vi "Werte ändern (DBL_8xZ.I._Rechteck) (SubVI).vi"(0 "geladene Werte (Zeit (s); Wert)":dbl[][](array[numeric]), 1 "Zykluslänge":dbl, 2 "Z.I.":string, 3 "Info":string, 4 "Format+Namen":string) -> (5 "Ausgang":dbl[][](array[numeric]) format="%.2f", 6 "Z.I.":string, 7 "Sperre":bool)   [LabVIEW 2010]
panel:
  out "Fehlermeldung":string="Zeit ist größer als Zykluslänge"
  in  "löschen":bool
  out "aktuel 8":dbl
  out "aktuel 7":dbl
  out "aktuel 6":dbl
  out "aktuel 5":dbl
  out "aktuel 4":dbl
  out "aktuel 3":dbl
  out "aktuel2":dbl
  out "Name 8":string
  in  "Numerisch 8":dbl
  out "Name 7":string
  in  "Numerisch 7":dbl
  out "Name 6":string
  in  "Numerisch 6":dbl
  out "Name 5":string
  in  "Numerisch 5":dbl
  out "Name 4":string
  in  "Numerisch 4":dbl
  out "Name 3":string
  in  "Numerisch 3":dbl
  out "Name 2":string
  in  "Numerisch 2":dbl
  out "aktuel1":dbl
  out "Name 1":string
  in  "Numerisch 1":dbl
  out "aktuell (Zeit (s); Wert)":dbl[][](array[numeric])
  out "XY Graph":T1(graph) caption="XY-Graph"
  out "Zykluslänge":dbl format="%.2f"
  out "Info":string
  in  "neue Werte (Zeit (s); Wert)":dbl[][](array[numeric])
  in  "ändern":bool
  in  "zurück":bool
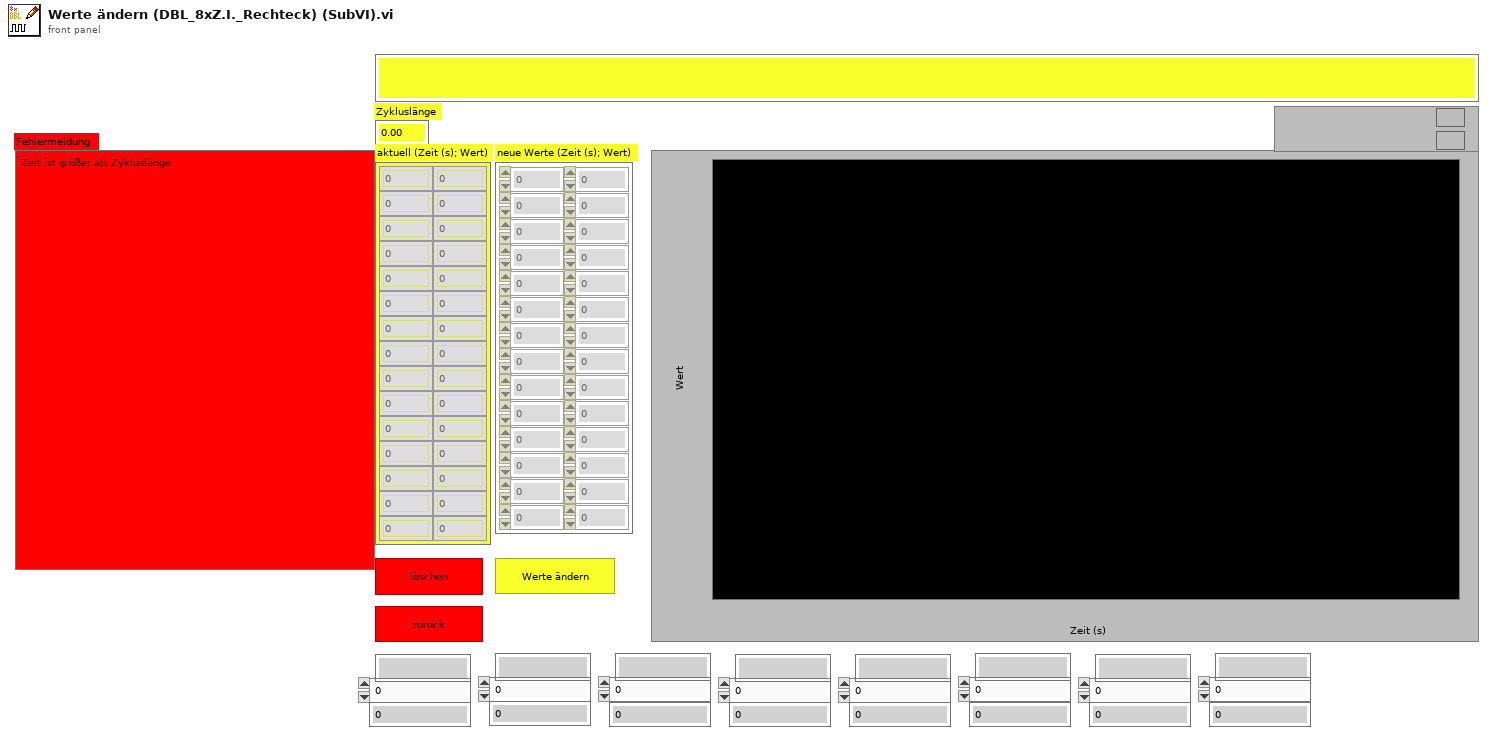
[diagram p1: front panel]
types:
  T1 = cluster{"neue Werte (Zeit (s); Wert)":dbl[], "neue Werte (Zeit (s); Wert)":dbl[]}[]
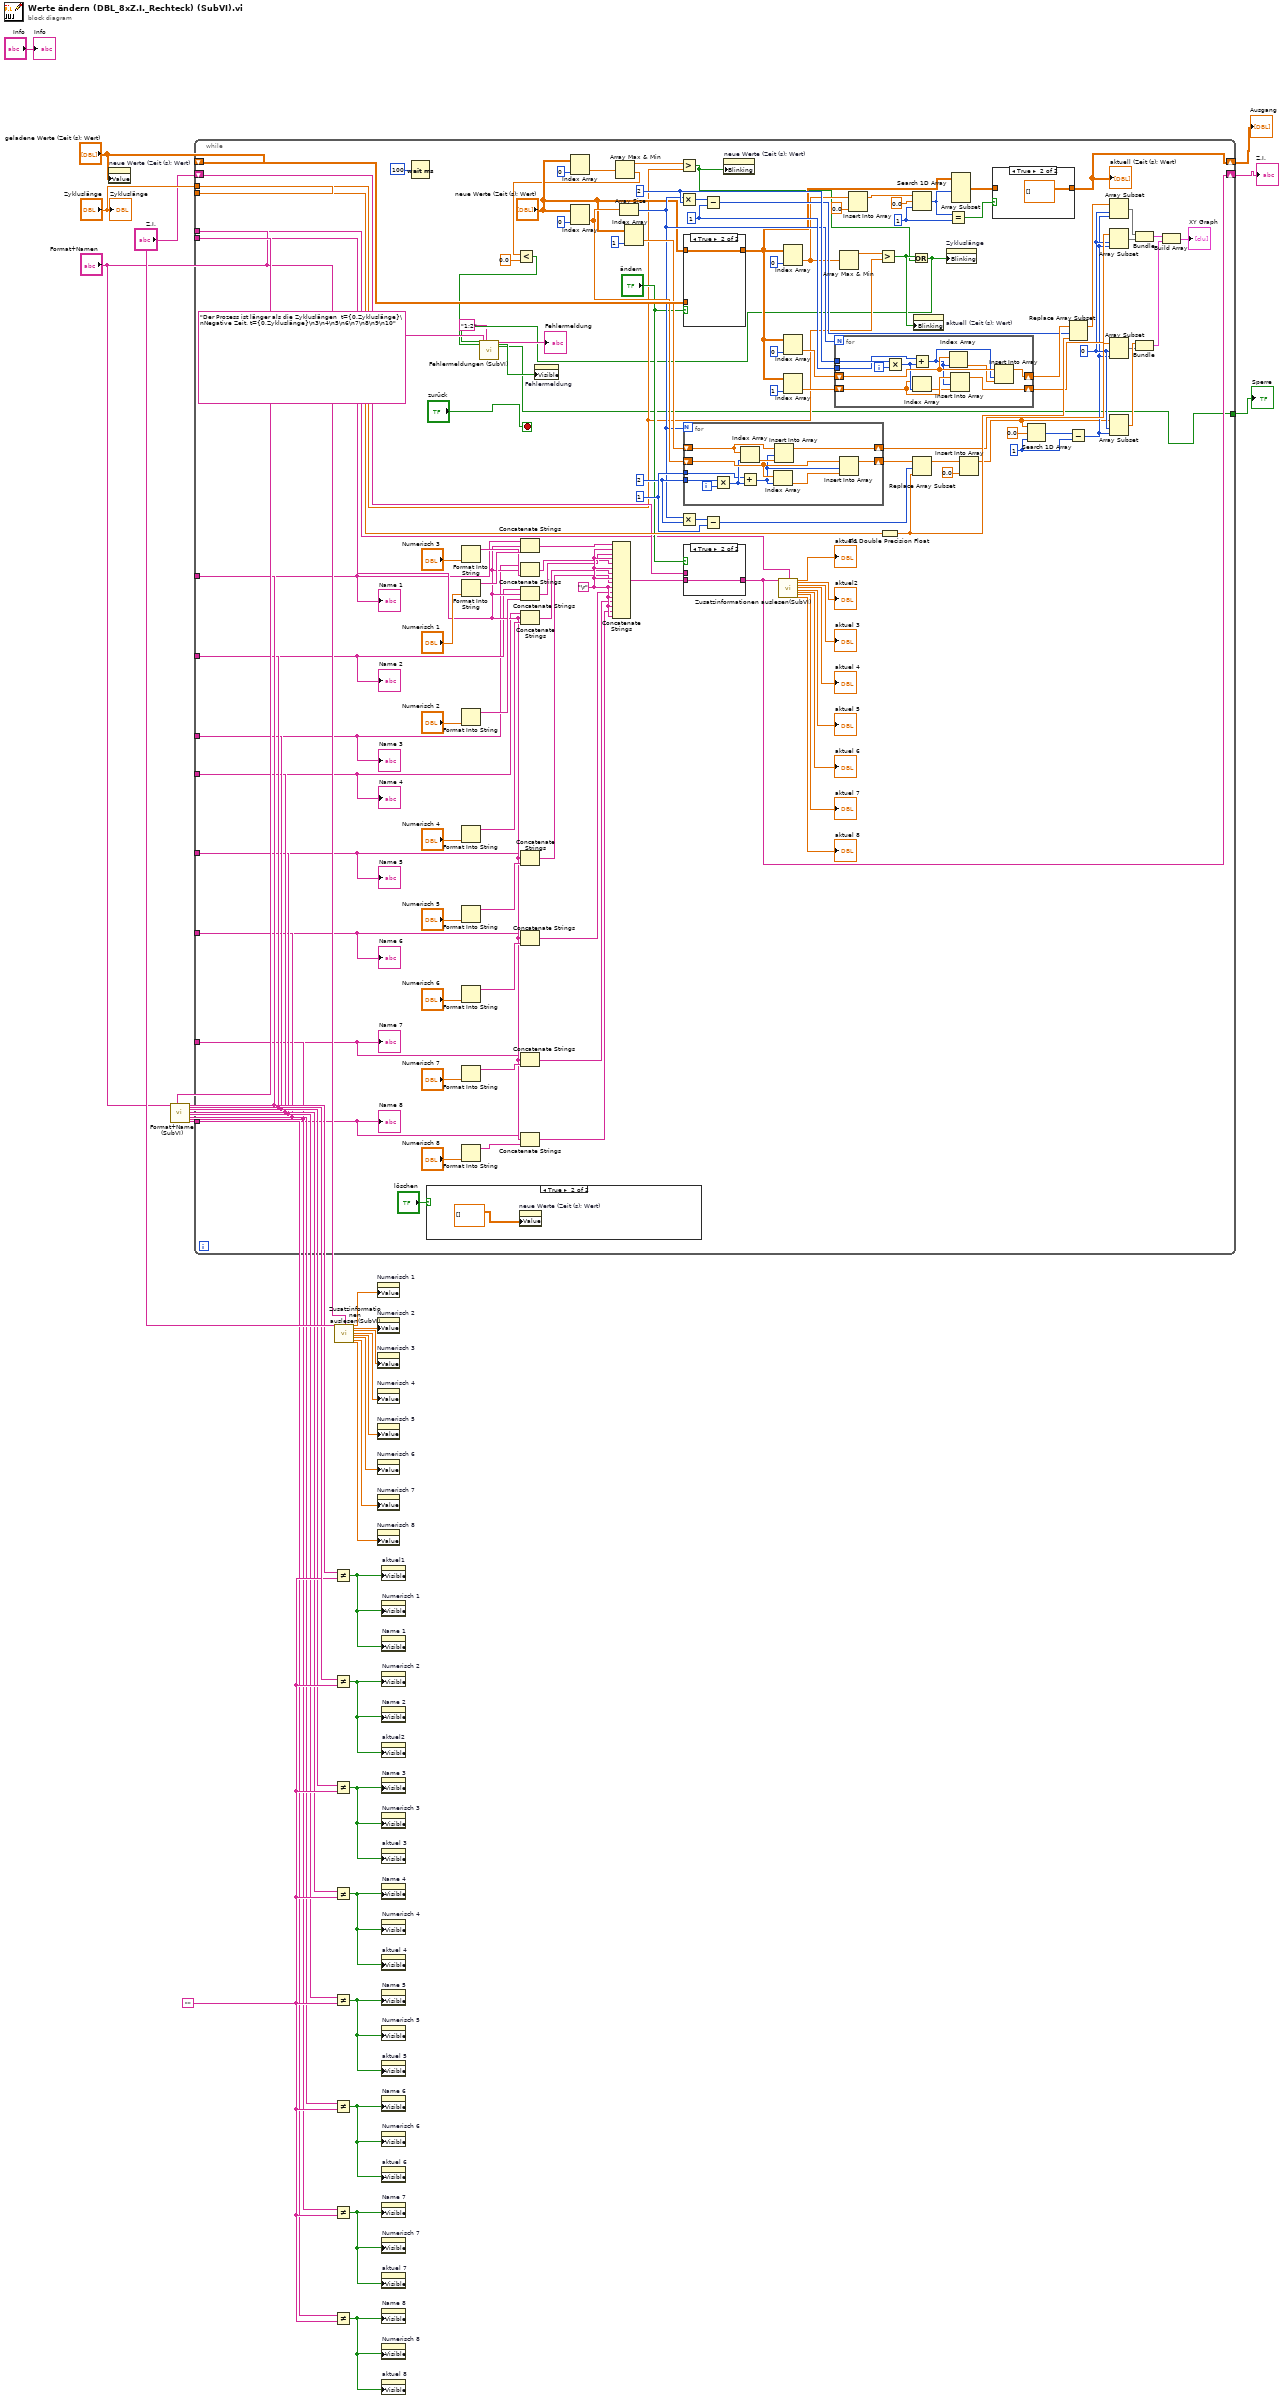
[diagram p0: block diagram]
diagram:
  w11 = ""
  n1 = property on="neue Werte (Zeit (s); Wert)" class="Arr (strikt)"("Value"="geladene Werte (Zeit (s); Wert)") -> ()  [unwired: 2 in, 2 out]
  n2 = call "Format+Name (SubVI).vi"("Format+Namen Eingang"="Format+Namen") -> ("Trennzeichen"=w31:string, "1"=w21:string, "2"=w18:string, "3"=w10:string, "4"=w9:string, "5"=w8:string, "6"=w7:string, "7"=w6:string, "8"=w5:string)  [unwired: 15 in, 3 out]
  n3 = while {
    shift-right: [w104] -> w2
    shift-left: "geladene Werte (Zeit (s); Wert)" -> [w151]
    tunnel: "Zykluslänge" -> [w47]
    tunnel: "Zykluslänge" -> [w141]
    shift-right: [w97] -> w1
    shift-left: "Z.I." -> [w102]
    tunnel: w21 -> [w56]
    tunnel: w31 -> [w80]
    tunnel: "Format+Namen" -> [w96]
    tunnel: w18 -> [w70]
    tunnel: w10 -> [w69]
    tunnel: w9 -> [w57]
    tunnel: w8 -> [w68]
    tunnel: w7 -> [w67]
    tunnel: w6 -> [w66]
    tunnel: w5 -> [w65]
    tunnel: [w35] -> w3
    stop <- "zurück" stop-if-true
    w79 = "\r"
    w105 = 1 ("Deaktivierter Index (Zeile)")
    w118 = 0 ("Index")
    w124 = 1 ("Startindex (0)")
    w136 = 1 ("y")
    w135 = 2 ("y")
    w143 = 1 ("y")
    w138 = 2 ("y")
    n4 = Wait (ms)(milliseconds to wait=u32 100 ("Zu wartende ms")) -> ()  [unwired: 1 out]
    n5 = case shown="True" "löschen" {
      frame False {
      }
      frame True {
        n6 = property on="neue Werte (Zeit (s); Wert)" class="Arr (strikt)"("Value"=dbl[][] [] ("neue Werte (Zeit (s); Wert)")) -> ()  [unwired: 2 in, 2 out]
      }
    }
    n7 = Format Into String("Numerisch 3") -> (resulting string=w91:string)  [unwired: 3 in, 1 out]
    n8 = Format Into String("Numerisch 1") -> (resulting string=w99:string)  [unwired: 3 in, 1 out]
    n9 = Format Into String("Numerisch 2") -> (resulting string=w94:string)  [unwired: 3 in, 1 out]
    n10 = Format Into String("Numerisch 4") -> (resulting string=w90:string)  [unwired: 3 in, 1 out]
    n11 = Format Into String("Numerisch 5") -> (resulting string=w87:string)  [unwired: 3 in, 1 out]
    n12 = Format Into String("Numerisch 6") -> (resulting string=w86:string)  [unwired: 3 in, 1 out]
    n13 = Format Into String("Numerisch 7") -> (resulting string=w83:string)  [unwired: 3 in, 1 out]
    n14 = Format Into String("Numerisch 8") -> (resulting string=w82:string)  [unwired: 3 in, 1 out]
    n15 = Concatenate Strings(w56, w80, w99) -> (w78:string)
    n16 = Concatenate Strings(w69, w80, w91) -> (w76:string)
    n17 = Concatenate Strings(w70, w80, w94) -> (w77:string)
    n18 = Concatenate Strings(w57, w80, w90) -> (w75:string)
    n19 = Concatenate Strings(w68, w80, w87) -> (w74:string)
    n20 = Concatenate Strings(w67, w80, w86) -> (w73:string)
    n21 = Concatenate Strings(w66, w80, w83) -> (w72:string)
    n22 = Concatenate Strings(w65, w80, w82) -> (w71:string)
    n23 = Index Array(array="neue Werte (Zeit (s); Wert)", index (col)=0 ("Deaktivierter Index (Spalte)")) -> (element=w48:dbl[])  [unwired: 1 in]
    n24 = Index Array(array="neue Werte (Zeit (s); Wert)", index (col)=0 ("Deaktivierter Index (Spalte)")) -> (element=w146:dbl[])  [unwired: 1 in]
    n25 = Concatenate Strings(w78, w79, w77, w79, w76, w79, w75, w79, w74, w79, w73, w79, w72, w79, w71, w79) -> (w98:string)
    n26 = Array Max & Min(array=w48) -> (max value=w50:dbl, min value=w39:dbl)  [unwired: 2 out]
    n27 = Less?(x=w39, y=0.0) -> (x < y?=w37:bool)
    n28 = Array Size(array=w146) -> (size(s)=w128:i32)
    n29 = Index Array(array="neue Werte (Zeit (s); Wert)", index (col)=1 ("Deaktivierter Index (Spalte)")) -> (element=w145:dbl[])  [unwired: 1 in]
    n30 = Greater?(x=w50, y=w47) -> (0:w45:bool)
    n31 = Multiply(x=w128, y=w135) -> (x*y=w137:i32)
    n32 = Multiply(x=w128, y=w138) -> (x*y=w144:i32)
    n33 = case shown="True" "ändern" {
      tunnel: w151 -> [w180 _]
      tunnel: [w180 w181] -> w107
      tunnel: "neue Werte (Zeit (s); Wert)" -> [_ w181]
      frame False {
      }
      frame True {
      }
    }
    n34 = for {
      N: w128 -> [_]
      shift-right: [w178] -> w126
      shift-left: w146 -> [w177]
      shift-right: [w173] -> w122
      shift-left: w145 -> [w175]
      tunnel: w138 -> [w170]
      tunnel: w143 -> [w169]
      i -> [w179]
      n35 = Multiply(x=w170, y=w179) -> (x*y=w176:i32)
      n36 = Index Array(array=w175, index=w176) -> (element=w174:dbl)
      n37 = Add(x=w169, y=w176) -> (x+y=w171:i32)
      n38 = Index Array(array=w177, index=w171) -> (element=w172:dbl)
      n39 = Insert Into Array(array=w175, index=w171, new element=w174) -> (w173:dbl[])
      n40 = Insert Into Array(array=w177, index=w171, new element=w172) -> (w178:dbl[])
    }
    n41 = case shown="True" "ändern" {
      tunnel: w102 -> [w154 _]
      tunnel: [w154 w155] -> w97
      tunnel: w98 -> [_ w155]
      frame False {
      }
      frame True {
      }
    }
    n42 = Subtract(x=w137, y=w136) -> (x-y=w133:i32)
    n43 = Subtract(x=w144, y=w143) -> (x-y=w142:i32)
    n44 = property on="neue Werte (Zeit (s); Wert)" class="Arr (strikt)"("Blinking"=w45) -> ()  [unwired: 2 in, 2 out]
    n45 = call "Zusatzinformationen auslesen(SubVI).vi"("Zusatzinformationen"=w97, "Format+Namen"=w96) -> ("1"=→"aktuel1":dbl, "2"=→"aktuel2":dbl, "3"=→"aktuel 3":dbl, "4"=→"aktuel 4":dbl, "5"=→"aktuel 5":dbl, "6"=→"aktuel 6":dbl, "7"=→"aktuel 7":dbl, "8"=→"aktuel 8":dbl)  [unwired: 18 in]
    n46 = Index Array(array=w107, index (col)=0 ("Deaktivierter Index (Spalte)")) -> (element=w53:dbl[])  [unwired: 1 in]
    n47 = Index Array(array=w107, index (col)=0 ("Deaktivierter Index (Spalte)")) -> (element=w130:dbl[])  [unwired: 1 in]
    n48 = Index Array(array=w107, index (col)=1 ("Deaktivierter Index (Spalte)")) -> (element=w129:dbl[])  [unwired: 1 in]
    n49 = for {
      N: w128 -> [_]
      shift-right: [w167] -> w134
      shift-left: w130 -> [w166]
      shift-right: [w162] -> w120
      shift-left: w129 -> [w164]
      tunnel: w135 -> [w159]
      tunnel: w136 -> [w158]
      i -> [w168]
      n50 = Multiply(x=w159, y=w168) -> (x*y=w165:i32)
      n51 = Add(x=w158, y=w165) -> (x+y=w160:i32)
      n52 = Index Array(array=w164, index=w165) -> (element=w163:dbl)
      n53 = Index Array(array=w166, index=w160) -> (element=w161:dbl)
      n54 = Insert Into Array(array=w164, index=w160, new element=w163) -> (w162:dbl[])
      n55 = Insert Into Array(array=w166, index=w160, new element=w161) -> (w167:dbl[])
    }
    n56 = Array Max & Min(array=w53) -> (max value=w52:dbl)  [unwired: 3 out]
    n57 = Insert Into Array(array=w53, new element=0.0 ("Neues Element/Teil-Array")) -> (w108:dbl[])  [unwired: 1 in]
    n58 = Greater?(x=w52, y=w47) -> (0:w46:bool)
    n59 = To Double Precision Float(number=w141) -> (double precision float=w132:dbl)
    n60 = Or(x=w46, y=w45) -> (x .or. y?=w41:bool)
    n61 = call "Fehlermeldungen (SubVI).vi"("Fehler 1"=w41, "Fehler 2"=w37, "Fehlermeldungen Namen"="Der Prozess ist länger als die Zykluslängen  t={0,Zykluslänge}\nNegative Zeit. t={0,Zykluslänge}\n3\n4\n5\n6\n7\n8\n9\n10", "Kritischefehler Positionen"="1;2") -> ("Fehlermeldung Ausgang"=→"Fehlermeldung":string, "Fehler?"=w42:bool, "Sperre"=w35:bool)  [unwired: 21 in]
    n62 = property on="Fehlermeldung" class="Str"("Visible"=w42) -> ()  [unwired: 2 in, 2 out]
    n63 = Search 1D Array(1D array=w108, element=0.0 ("Element"), start index (0)=w105) -> (index of element=w106:i32)
    n64 = Replace Array Subset(array=w126, new element=w132, index=w142) -> (w114:dbl[])
    n65 = property on="aktuell (Zeit (s); Wert)" class="Arr (strikt)"("Blinking"=w46) -> ()  [unwired: 2 in, 2 out]
    n66 = property on="Zykluslänge" class="DigWert (strikt)"("Blinking"=w41) -> ()  [unwired: 2 in, 2 out]
    n67 = Equal?(x=w106, y=w105) -> (x = y?=w55:bool)
    n68 = Array Subset(array=w107, length (row)=w106) -> (w103:dbl[][])  [unwired: 3 in]
    n69 = Insert Into Array(array=w114, new element=0.0 ("Neues Element/Teil-Array")) -> (w113:dbl[])  [unwired: 1 in]
    n70 = case shown="True" w55 {
      tunnel: [w156 dbl[][] [] ("neue Werte (Zeit (s); Wert)")] -> w104
      tunnel: w103 -> [w156 _]
      frame False {
      }
      frame True {
      }
    }
    "aktuell (Zeit (s); Wert)" <- w104
    n71 = Search 1D Array(1D array=w113, element=0.0 ("Element"), start index (0)=w124) -> (index of element=w125:i32)
    n72 = Replace Array Subset(array=w134, new element=w132, index=w133) -> (w116:dbl[])
    n73 = Subtract(x=w125, y=w124) -> (x-y=w117:i32)
    n74 = Array Subset(array=w116, index=w118, length=w117) -> (w115:dbl[])
    n75 = Array Subset(array=w120, index=w118, length=w117) -> (w119:dbl[])
    n76 = Array Subset(array=w122, index=w118, length=w117) -> (w121:dbl[])
    n77 = Array Subset(array=w113, index=w118, length=w117) -> (w123:dbl[])
    n78 = Bundle(w115, w119) -> (w131:cluster{dbl[], dbl[]})  [unwired: 1 in]
    n79 = Bundle(w123, w121) -> (w139:cluster{dbl[], dbl[]})  [unwired: 1 in]
    n80 = Build Array(w131, w139) -> (→"XY Graph":cluster{dbl[], dbl[]}[])
    "Name 1" <- w56
    "Name 2" <- w70
    "Name 3" <- w69
    "Name 4" <- w57
    "Name 5" <- w68
    "Name 6" <- w67
    "Name 7" <- w66
    "Name 8" <- w65
  }
  "Sperre" <- w3
  "Ausgang" <- w2
  "Z.I." <- w1
  n81 = Not Equal?(x=w21, y=w11) -> (x != y?=w20:bool)
  n82 = Not Equal?(x=w18, y=w11) -> (x != y?=w19:bool)
  n83 = Not Equal?(x=w10, y=w11) -> (x != y?=w17:bool)
  n84 = Not Equal?(x=w9, y=w11) -> (x != y?=w16:bool)
  n85 = Not Equal?(x=w8, y=w11) -> (x != y?=w15:bool)
  n86 = Not Equal?(x=w7, y=w11) -> (x != y?=w14:bool)
  n87 = Not Equal?(x=w6, y=w11) -> (x != y?=w13:bool)
  n88 = Not Equal?(x=w5, y=w11) -> (x != y?=w12:bool)
  n89 = call "Zusatzinformationen auslesen(SubVI).vi"("Zusatzinformationen"="Z.I.", "Format+Namen"="Format+Namen") -> ("1"=w29:dbl, "2"=w28:dbl, "3"=w27:dbl, "4"=w26:dbl, "5"=w25:dbl, "6"=w24:dbl, "7"=w23:dbl, "8"=w22:dbl)  [unwired: 18 in]
  n90 = property on="Numerisch 1" class="DigWert (strikt)"("Value"=w29) -> ()  [unwired: 2 in, 2 out]
  n91 = property on="Numerisch 2" class="DigWert (strikt)"("Value"=w28) -> ()  [unwired: 2 in, 2 out]
  n92 = property on="Numerisch 3" class="DigWert (strikt)"("Value"=w27) -> ()  [unwired: 2 in, 2 out]
  n93 = property on="Numerisch 4" class="DigWert (strikt)"("Value"=w26) -> ()  [unwired: 2 in, 2 out]
  n94 = property on="Numerisch 5" class="DigWert (strikt)"("Value"=w25) -> ()  [unwired: 2 in, 2 out]
  n95 = property on="Numerisch 6" class="DigWert (strikt)"("Value"=w24) -> ()  [unwired: 2 in, 2 out]
  n96 = property on="Numerisch 7" class="DigWert (strikt)"("Value"=w23) -> ()  [unwired: 2 in, 2 out]
  n97 = property on="Numerisch 8" class="DigWert (strikt)"("Value"=w22) -> ()  [unwired: 2 in, 2 out]
  n98 = property on="aktuel1" class="DigWert (strikt)"("Visible"=w20) -> ()  [unwired: 2 in, 2 out]
  n99 = property on="Numerisch 1" class="DigWert (strikt)"("Visible"=w20) -> ()  [unwired: 2 in, 2 out]
  n100 = property on="Name 1" class="Str"("Visible"=w20) -> ()  [unwired: 2 in, 2 out]
  n101 = property on="Numerisch 2" class="DigWert (strikt)"("Visible"=w19) -> ()  [unwired: 2 in, 2 out]
  n102 = property on="Name 2" class="Str"("Visible"=w19) -> ()  [unwired: 2 in, 2 out]
  n103 = property on="aktuel2" class="DigWert (strikt)"("Visible"=w19) -> ()  [unwired: 2 in, 2 out]
  n104 = property on="Name 3" class="Str"("Visible"=w17) -> ()  [unwired: 2 in, 2 out]
  n105 = property on="Numerisch 3" class="DigWert (strikt)"("Visible"=w17) -> ()  [unwired: 2 in, 2 out]
  n106 = property on="aktuel 3" class="DigWert (strikt)"("Visible"=w17) -> ()  [unwired: 2 in, 2 out]
  n107 = property on="Name 4" class="Str"("Visible"=w16) -> ()  [unwired: 2 in, 2 out]
  n108 = property on="Numerisch 4" class="DigWert (strikt)"("Visible"=w16) -> ()  [unwired: 2 in, 2 out]
  n109 = property on="aktuel 4" class="DigWert (strikt)"("Visible"=w16) -> ()  [unwired: 2 in, 2 out]
  n110 = property on="Name 5" class="Str"("Visible"=w15) -> ()  [unwired: 2 in, 2 out]
  n111 = property on="Numerisch 5" class="DigWert (strikt)"("Visible"=w15) -> ()  [unwired: 2 in, 2 out]
  n112 = property on="aktuel 5" class="DigWert (strikt)"("Visible"=w15) -> ()  [unwired: 2 in, 2 out]
  n113 = property on="Name 6" class="Str"("Visible"=w14) -> ()  [unwired: 2 in, 2 out]
  n114 = property on="Numerisch 6" class="DigWert (strikt)"("Visible"=w14) -> ()  [unwired: 2 in, 2 out]
  n115 = property on="aktuel 6" class="DigWert (strikt)"("Visible"=w14) -> ()  [unwired: 2 in, 2 out]
  n116 = property on="Name 7" class="Str"("Visible"=w13) -> ()  [unwired: 2 in, 2 out]
  n117 = property on="Numerisch 7" class="DigWert (strikt)"("Visible"=w13) -> ()  [unwired: 2 in, 2 out]
  n118 = property on="aktuel 7" class="DigWert (strikt)"("Visible"=w13) -> ()  [unwired: 2 in, 2 out]
  n119 = property on="Name 8" class="Str"("Visible"=w12) -> ()  [unwired: 2 in, 2 out]
  n120 = property on="Numerisch 8" class="DigWert (strikt)"("Visible"=w12) -> ()  [unwired: 2 in, 2 out]
  n121 = property on="aktuel 8" class="DigWert (strikt)"("Visible"=w12) -> ()  [unwired: 2 in, 2 out]
  "Info" <- "Info"
  "Zykluslänge" <- "Zykluslänge"
